vi "init.vi"(8 "error in (no error)":errorcluster, 11 "LoopInternalConfig in":refnum<class "LoopInternalConfig.lvclass">) -> (0 "error out":errorcluster, 3 "LoopInternalConfig out":refnum<class "LoopInternalConfig.lvclass">)   [LabVIEW 2013, in "ComponentData.lvlib" / "LoopInternalConfig.lvclass"]
uses:
  <userlib>/Common/Component/common_application/RT/ComponentData/ConfigurationHandler/LoopInternalConfig/LoopInternalConfig.lvclass
  <userlib>/Common/Component/common_application/MyComputer/ComponentConfiguration/ComponentConfigurationTypedefs/loopInternalConfig.ctl
  <userlib>/Common/Component/common_application/RT/ComponentData/ConfigurationHandler/LoopInternalConfig/LoopInternalConfig.lvclass/LoopInternalConfig.ctl
  <vilib>/Utility/xml.llb/Read From XML File(string).vi
  <userlib>/Common/Component/common_application/MyComputer/ComponentConfiguration.lvlib
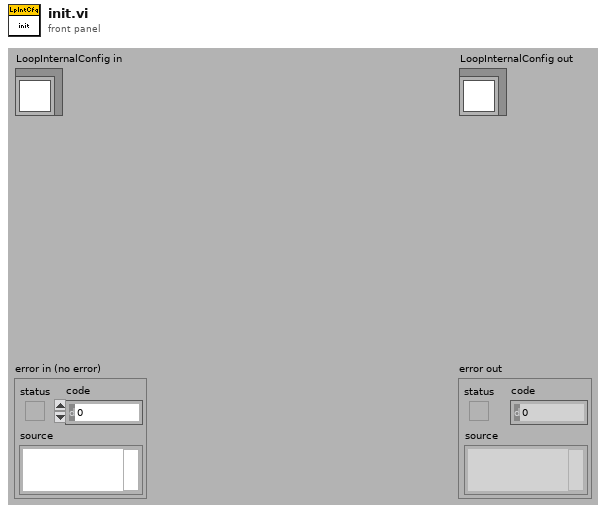
[diagram p1: front panel]
types:
  T1 = typedef "ComponentConfiguration.lvlib/loopInternalConfig.ctl" = cluster{"fpgaClockSpeed_Hz":dbl}
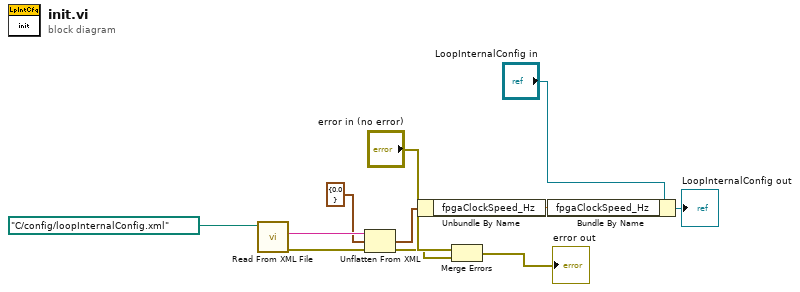
[diagram p0: block diagram]
diagram:
  n1 = call-poly <vilib>:"Read From XML File.vi"("XML File Path"=path "C:/config/loopInternalConfig.xml" ("configuration file path")) -> ("error out"=w4:errorcluster, "XML Elements"=w8:string)  [unwired: 8 in, 1 out]
  n2 = Unflatten From XML(xml string=w8, type=T1 {"fpgaClockSpeed_Hz"=0.0} ("loopInternalConfig"), error in (no error)=w4) -> (value=w6:T1, error out=w2:errorcluster)
  n3 = Unbundle By Name(w6) -> ("fpgaClockSpeed_Hz"=w5:dbl)
  n4 = Merge Errors("error in (no error)", w2) -> (→"error out":errorcluster)
  n5 = Bundle By Name(cluster="LoopInternalConfig in", "fpgaClockSpeed_Hz"=w5) -> (→"LoopInternalConfig out":refnum<class "LoopInternalConfig.lvclass">)
